vi "CAPTH-Init Data.vi"(0 "Freqs":dbl[](array[numeric]), 5 "EAR":i32(ring), 7 "Folder":path, 11 "error in (no error)":errorcluster) -> (4 "data array":cluster{"Freqs":dbl[], dbl[], "Max SPL":dbl[]}[](array[cluster]), 15 "error out":errorcluster)   [LabVIEW 2020]
uses:
  epl-vi-lib/Utility VIs/Type Defs/Speaker ring.ctl
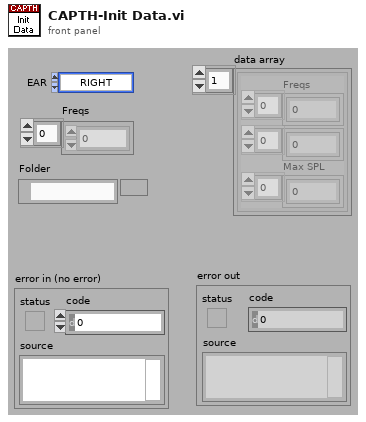
[diagram p1: front panel]
types:
  T1 = typedef "Speaker ring.ctl" = enum16{"Right primary", "Right secondary", "Left primary", "Left secondary"}
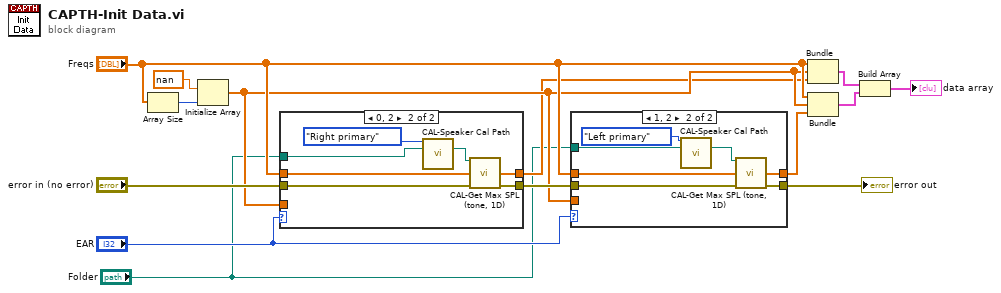
[diagram p0: block diagram]
diagram:
  n1 = Array Size(array="Freqs") -> (size(s)=w14:i32)
  n2 = Initialize Array(nan ("element"), w14) -> (w8:dbl[])
  n3 = case shown="0, 2" "EAR" {
    tunnel: "Freqs" -> [_ w17]
    tunnel: [w16 w23] -> w4
    tunnel: w8 -> [w16 _]
    tunnel: "error in (no error)" -> [w15 w22]
    tunnel: [w15 w21] -> w11
    tunnel: "Folder" -> [_ w19]
    frame 1, Default {
    }
    frame 0, 2 {
      n4 = call "CAL-Speaker Cal Path.vi"("Speaker"=Speaker_ring."Right primary", "Data Folder"=w19) -> ("Cal Path"=w18:path)  [unwired: 12 in, 1 out]
      n5 = call "CAL-Get Max SPL (tone, 1D).vi"("Speaker name"=w18, "Frequency (kHz)"=w17, "error in (no error)"=w22) -> ("Max SPL"=w23:dbl[], "error out"=w21:errorcluster)  [unwired: 11 in]
    }
  }
  n6 = case shown="1, 2" "EAR" {
    tunnel: [w25 w32] -> w7
    tunnel: w11 -> [w24 w31]
    tunnel: "Freqs" -> [_ w26]
    tunnel: w8 -> [w25 _]
    tunnel: [w24 w30] -> w2
    tunnel: "Folder" -> [_ w28]
    frame 0, Default {
    }
    frame 1, 2 {
      n7 = call "CAL-Speaker Cal Path.vi"("Speaker"=Speaker_ring."Left primary", "Data Folder"=w28) -> ("Cal Path"=w27:path)  [unwired: 12 in, 1 out]
      n8 = call "CAL-Get Max SPL (tone, 1D).vi"("Speaker name"=w27, "Frequency (kHz)"=w26, "error in (no error)"=w31) -> ("Max SPL"=w32:dbl[], "error out"=w30:errorcluster)  [unwired: 11 in]
    }
  }
  "error out" <- w2
  n9 = Bundle("Freqs"="Freqs", w8, "Max SPL"=w4) -> (w6:cluster{"Freqs":dbl[], dbl[], "Max SPL":dbl[]})  [unwired: 1 in]
  n10 = Bundle("Freqs"="Freqs", w8, "Max SPL"=w7) -> (w5:cluster{"Freqs":dbl[], dbl[], "Max SPL":dbl[]})  [unwired: 1 in]
  n11 = Build Array(w6, w5) -> (→"data array":cluster{"Freqs":dbl[], dbl[], "Max SPL":dbl[]}[])
